vi "Global Variables.vi"() -> ()   [LabVIEW 2013]
panel:
  in  "Inkscape ratio":dbl
  out "Simulation Stop":bool=TRUE
  in  "Amplifier Setting":dbl=-10.0
  in  "Read Tip Voltage":dbl
  out "Read data":bool=TRUE
  in  "Old Y Offset":dbl
  in  "Old X Offset":dbl
  in  "Y Offset":dbl
  in  "X Offset":dbl
  in  "Old Image Width":dbl=40.0
  in  "Old Image Height":dbl=40.0
  in  "Image Width":dbl=40.0
  in  "Image Height":dbl=40.0
  in  "Old RGB Value":u32
  in  "RGB Value":u32
  in  "Old Visible":bool=TRUE
  in  "Visible":bool=TRUE
  in  "Old Center of Vision":string="(0,0,0)"
  in  "Center of Vision":string="(0,0,0)"
  in  "Old Wire Width":dbl=0.01
  in  "Old Voltage":dbl
  in  "Old Y":dbl=15.0
  in  "Old X":dbl=15.0
  in  "Wire Width":dbl=0.1
  in  "Voltage":dbl
  in  "Y":dbl=7.418777765268947
  in  "X":dbl=26.509542
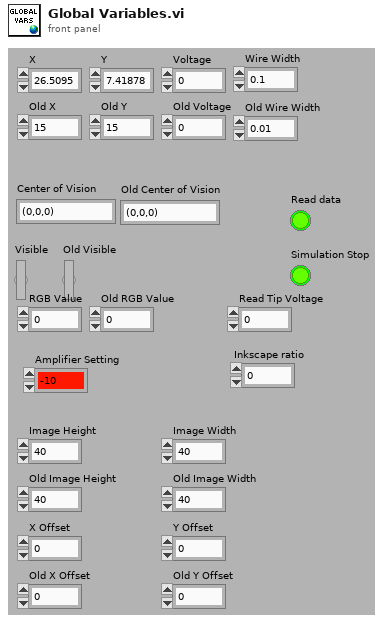
[diagram p1: front panel]
diagram:
